vi "moving average.vi"() -> ()   [LabVIEW 2017]
panel:
  in  "window size":i32=5
  in  "X":dbl[](array[numeric])
  out "averaged X":dbl[](array[numeric])
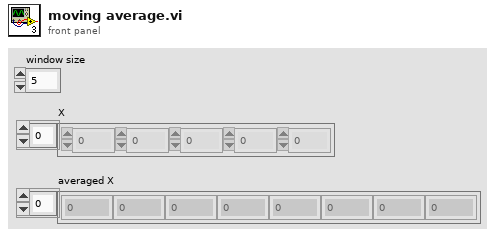
[diagram p1: front panel]
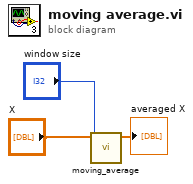
[diagram p0: block diagram]
diagram:
  n1 = call "moving_average.vi"("window size"="window size", "X"="X") -> ("averaged X"=→"averaged X":dbl[])  [unwired: 9 in]
